vi "E-Stop Present.vi"(8 "error in":errorcluster, 11 "Light Stack in":refnum<class "Light Stack.lvclass">) -> (0 "error out":errorcluster, 3 "Light Stack out":refnum<class "Light Stack.lvclass">)   [LabVIEW 2018, in "Light Stack.lvlib" / "Light Stack.lvclass"]
uses:
  Light Stack.lvclass
  Light Stack.lvclass/Light Stack.ctl
  Custom Controls/Light Select.ctl
  Custom Controls/Light Mode.ctl
  Light Stack.lvlib
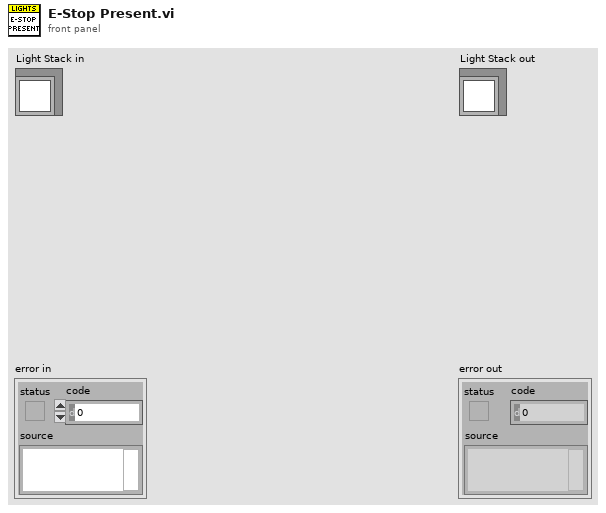
[diagram p1: front panel]
types:
  T1 = typedef "Light Stack.lvlib/Light Select.ctl" = enum16{"Red", "Amber", "Green", "Blue"}
  T2 = typedef "Light Stack.lvlib/Light Mode.ctl" = enum16{"OFF", "ON", "BLINK"}
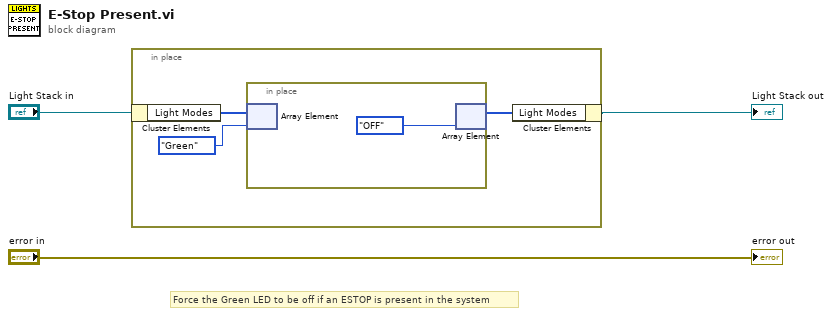
[diagram p0: block diagram]
diagram:
  # "Force the Green LED to be off if an ESTOP is present in the system"
  n1 = in-place {
    n2 = in-place-cluster #1("Light Stack in") -> ("Light Modes"=w6:T2[])
    n3 = in-place {
      n4 = in-place-array #2(w6, Light_Select."Green" ("Light Select")) -> ()  [unwired: 1 out]
      n5 = in-place-array #2(Light_Mode."OFF" ("Light Mode")) -> (w4:T2[])  [unwired: 1 out]
    }
    n6 = in-place-cluster #1("Light Modes"=w4) -> (→"Light Stack out":refnum<class "Light Stack.lvclass">)
  }
  "error out" <- "error in"
